vi "Set Virt Instr.vi"(8 "error in (no error)":errorcluster, 10 "Virt Instr":T1(c390), 11 "MSS in":refnum<class "Measure and Stimulus Subsystems.lvclass">) -> (0 "error out":errorcluster, 3 "MSS out":refnum<class "Measure and Stimulus Subsystems.lvclass">)   [LabVIEW 2023, in "HAL GOOP4.lvlib" / "Measure and Stimulus Subsystems.lvclass"]
uses:
  Measure and Stimulus Subsystems.lvclass
  Virt Instr Host/Virt Instr Local.lvclass
  Measure and Stimulus Subsystems.lvclass/Measure and Stimulus Subsystems.ctl
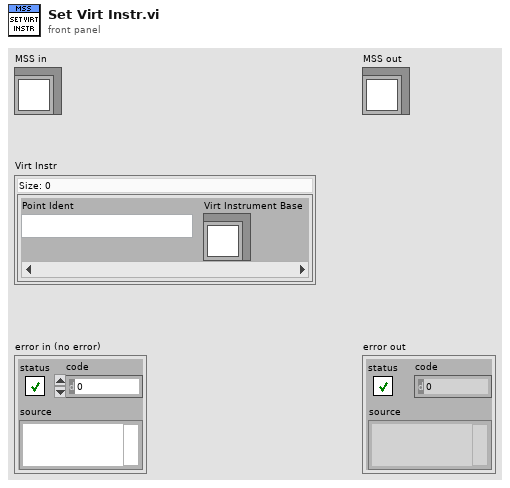
[diagram p1: front panel]
types:
  T1 = map{string, refnum<class "Virt Instr Local.lvclass">}
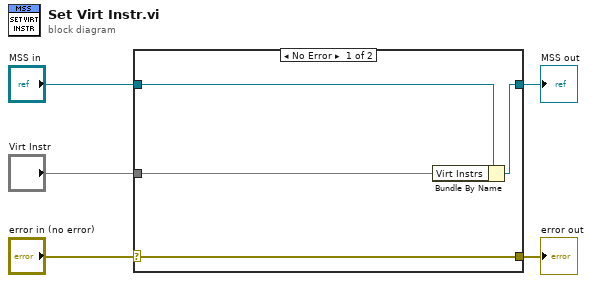
[diagram p0: block diagram]
diagram:
  n1 = case shown="No Error" "error in (no error)" {
    selector: "error in (no error)" -> [w9 w10]
    tunnel: [w9 w10] -> w4
    tunnel: [w7 w11] -> w2
    tunnel: "MSS in" -> [w8 w11]
    tunnel: "Virt Instr" -> [w6 _]
    frame No Error {
      n2 = Bundle By Name(cluster=w8, "Virt Instrs"=w6) -> (w7:refnum<class "Measure and Stimulus Subsystems.lvclass">)
    }
    frame Error {
    }
  }
  "error out" <- w4
  "MSS out" <- w2
